vi "Constructor_ZeroMQ_Context.vi"(8 "error in":errorcluster, 11 "dll":path) -> (0 "error out":errorcluster, 3 "context out":refnum<class "Context.lvclass">)   [LabVIEW 2025, in "ZeroMQ.lvlib" / "Context.lvclass"]
doc: "Instantiate ZeroMQ and return a <b>context</b> to create sockets with. Ideally, this should only be called once per application and the context shared.\n\nPreviously called <b>zmq_init</b>.\n\nDetailed API documentation: http://api.zeromq.org/3-2:zmq-ctx-new"
uses:
  Context.lvclass
  Context.lvclass/Context.ctl
  libzmq-v143-mt-4_3_6/LibZMQ.lvlib
panel:
  # "ØMQ"
  # "labview"
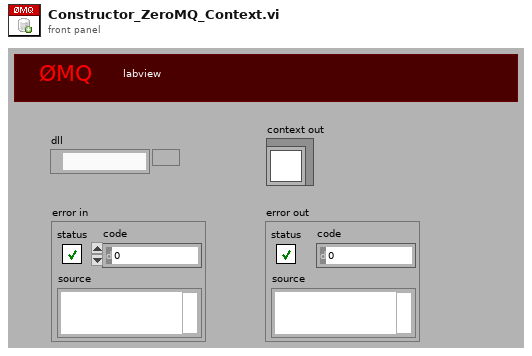
[diagram p1: front panel]
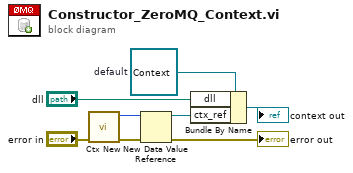
[diagram p0: block diagram]
diagram:
  w8 = refnum<class "Context.lvclass"> refnum  # default
  n1 = call "Ctx New.vi"("error in (no error)"="error in") -> ("error out"=w2:errorcluster, "function return"=w3:u64)  [unwired: 9 in]
  n2 = New Data Value Reference(data value=w3, error in=w2) -> (data value reference=w6:refnum<data-value>, error out=→"error out":errorcluster)
  n3 = Bundle By Name(cluster=w8, "dll"="dll", "ctx_ref"=w6) -> (→"context out":refnum<class "Context.lvclass">)
